vi "Read Device State.vi"(8 "error in (no error)":errorcluster, 10 "Device Command":T1(ring), 11 "VISA resource name":refnum<visa-resource-name>) -> (0 "error out":errorcluster, 1 "Device Reply":enum16{"Off", "On"}(ring), 2 "Device Command":T1(ring), 3 "VISA resource name out":refnum<visa-resource-name>)   [LabVIEW 2010, in "Temptronic TP04300.lvlib"]
doc: "This VI writes a device specific query and reads the intrument reply, indicating its state.\n\nThe following querries are supported:\n\n<b>Air Flow</b> - returns whether the main air flow is On or Off.\n\n Returns Command Argument \n = 0 the air flow is off\n = 1 the air flow is on\n\n<b>Trickle Flow</b> - returns whether the trickle air flow is On or Off.\n\n Returns Command Argument \n = 0 the trickle flow is off\n = 1 the trickle flow is on\n \n<b>Head</b> - returns whether the head is Up or Down position.\n\n Returns Command Argument \n = 0 the head is in Up position\n = 1 the head Down is in Down position\n\n<b>Head Lock</b> - returns the head lock/unlock state.\n\n Returns Command Argument \n = 0 the head is unlocked\n = 1 the head is locked\n\n<b>Compressor</b> - returns whether the compressor is On or Off.\n\n Returns Command Argument \n = 0 the compressor is off\n = 1 the compressor is on"
uses:
  Temptronic TP04300.lvlib
  Instance           1 25Saved   Read Device State .vi
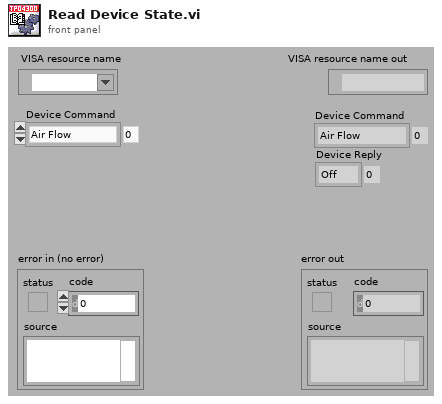
[diagram p1: front panel]
types:
  T1 = enum16{"Air Flow", "Trickle Flow", "Head", "Head Lock", "Compressor"}
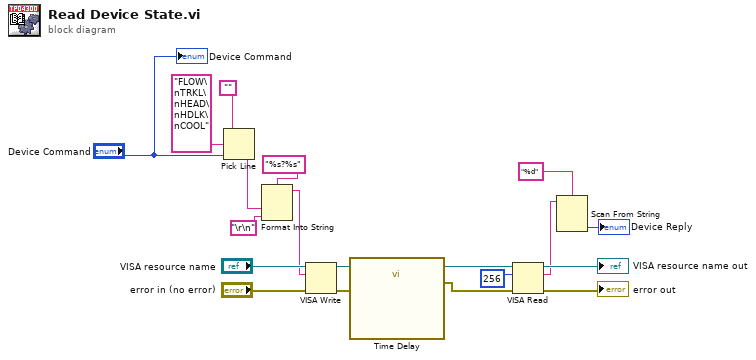
[diagram p0: block diagram]
diagram:
  n1 = Pick Line(string ("")="", multi-line string="FLOW\nTRKL\nHEAD\nHDLK\nCOOL", line index="Device Command") -> (output string=w14:string)
  n2 = Format Into String(format string="%s?%s", w14, "\r\n") -> (resulting string=w12:string)  [unwired: 2 in, 1 out]
  n3 = VISA Write(VISA resource name="VISA resource name", write buffer=w12, error in (no error)="error in (no error)") -> (VISA resource name out=w10:refnum<visa-resource-name>, error out=w2:errorcluster)  [unwired: 1 out]
  n4 = call "Time Delay"("error in (no error)"=w2) -> ("error out"=w1:errorcluster)  [unwired: 10 in]
  n5 = VISA Read(VISA resource name=w10, byte count=u32 256, error in (no error)=w1) -> (VISA resource name out=→"VISA resource name out":refnum<visa-resource-name>, read buffer=w4:string, error out=→"error out":errorcluster)  [unwired: 1 out]
  n6 = Scan From String(format string="%d", input string=w4) -> (output 1=→"Device Reply":enum16{"Off", "On"})  [unwired: 3 in, 3 out]
  "Device Command" <- "Device Command"
